vi "SortEngineer.vi"(7 "Invert?":bool, 8 "error in (no error)":errorcluster, 11 "Array in":T1[](array[typedef])) -> (0 "error out":errorcluster, 3 "Array out":T1[](array[typedef]))   [LabVIEW 2017, in "Client.lvlib" / "ParserSorter.lvlib"]
doc: "Check If Days Open > 0,1 and calculate Score based on Prio specific Base Values"
uses:
  ParserSorter.lvlib
  SR Data.ctl
  AE Group.ctl
  SR Status.ctl
  SR Level.ctl
  SR Type.ctl
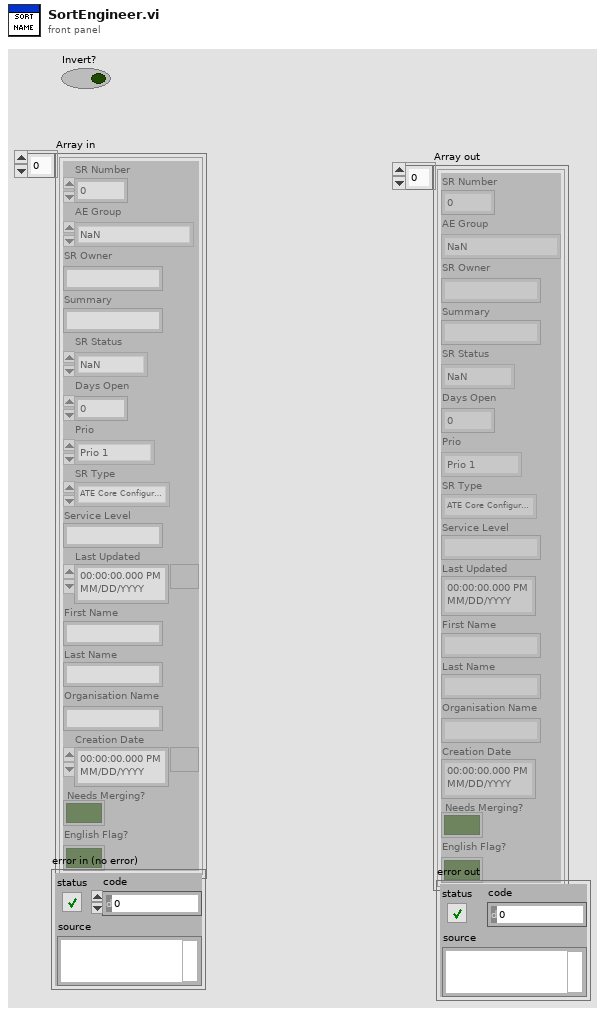
[diagram p1: front panel]
types:
  T1 = typedef "Client.lvlib/ParserSorter.lvlib/SR Data.ctl" = cluster{"SR Number":i64, "AE Group":T2, "SR Owner":string, "Summary":string, "SR Status":T3, "Days Open":dbl, "Prio":T4, "SR Type":T5, "Service Level":string, "Last Updated":timestamp, "First Name":string, "Last Name":string, "Organisation Name":string, "Creation Date":timestamp, "Needs Merging?":bool, "English Flag?":bool}
  T2 = typedef "Client.lvlib/ParserSorter.lvlib/AE Group.ctl" = enum32{"NaN", "AE-Germany", "AE-Poland", "AE-Switzerland", "AE-Czech Republic", "AE-Hungary", "AE-Romania", "AE-Slovakia", "AE-Slovenia"}
  T3 = typedef "Client.lvlib/ParserSorter.lvlib/SR Status.ctl" = enum32{"NaN", "Caller Abandoned", "Created in Error", "Declined to Purchase Support", "Expired", "Forum Resolved AE", "Forum Resolved Customer", "IN WORK", "IN WORK Collab with AES", "IN WORK Collab with PSE", "IN WORK Collab with SE", "IN WORK Escalation", "IN WORK Customer Added Note", "Open", "Potentially Resolved", "POC Resolved", "Resolved", "RMA Waiting on Customer", "RMA Open", "RMA In Progress", "RMA Closed - DOA", "RMA Closed", "RMA Approved for Return", "Project Complete", "Presumed Resolved", "IN WORK Wait on Customer"}
  T4 = typedef "Client.lvlib/ParserSorter.lvlib/SR Level.ctl" = enum16{"Prio 1", "Prio 2", "Prio 3", "Prio 4"}
  T5 = typedef "Client.lvlib/ParserSorter.lvlib/SR Type.ctl" = enum32{"NaN", "ATE Core Configurations (BYOATE)", "Activation", "BioBench", "CAN", "CM C Series", "Calibration", "Consulting Services", "CounterTimer", "DAQExpress", "DASYLab", "DIAdem", "DMM", "DSA HW", "Digital_IO", "FIRST (NIC Only)", "FieldBus", "FieldPoint", "Functional Savety", "GATI", "GPIB", "HMI and Industrial PCs", "HiQ", "HighSpeedDigital_IO", "IMAQ", "IOTech Vibration", "Industrial Communications", "InsightCM", "LV", "LV CD&Sim", "LV Comms", "LV Controls Add-Ons", "LV Embedded", "LV MathScript RT", "LV NXG", "LV NXT", "LVDSC", "LVFPGA", "LVPDA and LV Touch Panel", "LVRT", "LabWindows_CVI", "Lookout", "MATRIXx", "MStudioDotNet", "MStudioVisualBasic", "MStudioVisualC", "Measure (Legacy)", "Motion", "MultifunctionDAQ", "Multimedia Test HW/SW", "Multisim (EWB)", "NI Update Service", "OPC Servers", "Optical (OSI)", "PXI Controllers, Chassis, MXI", "PXI Timing and Sync", "Power Supplies and SMUs", "Powertrain Controls", "RAID", "RF", "RF Software", "RIO", "SC Express", "SCC", "SCXI", "SPEEDY-33 (Hyperception)", "STS", "ScopeDigitizers", "Serial", "Signal Sources", "SignalCondOther", "SignalExpress", "Software Defined Intruments", "Sound and Vibration SW", "Switch Executive", "Switches", "TestStand", "USRP", "Ultiboard (EWB)", "VBench", "VI Logger", "VXI_MXI", "VeriStand", "VisionSW", "VolumeLicenseMgr", "WSN", "Web UI Builder", "myRIO"}
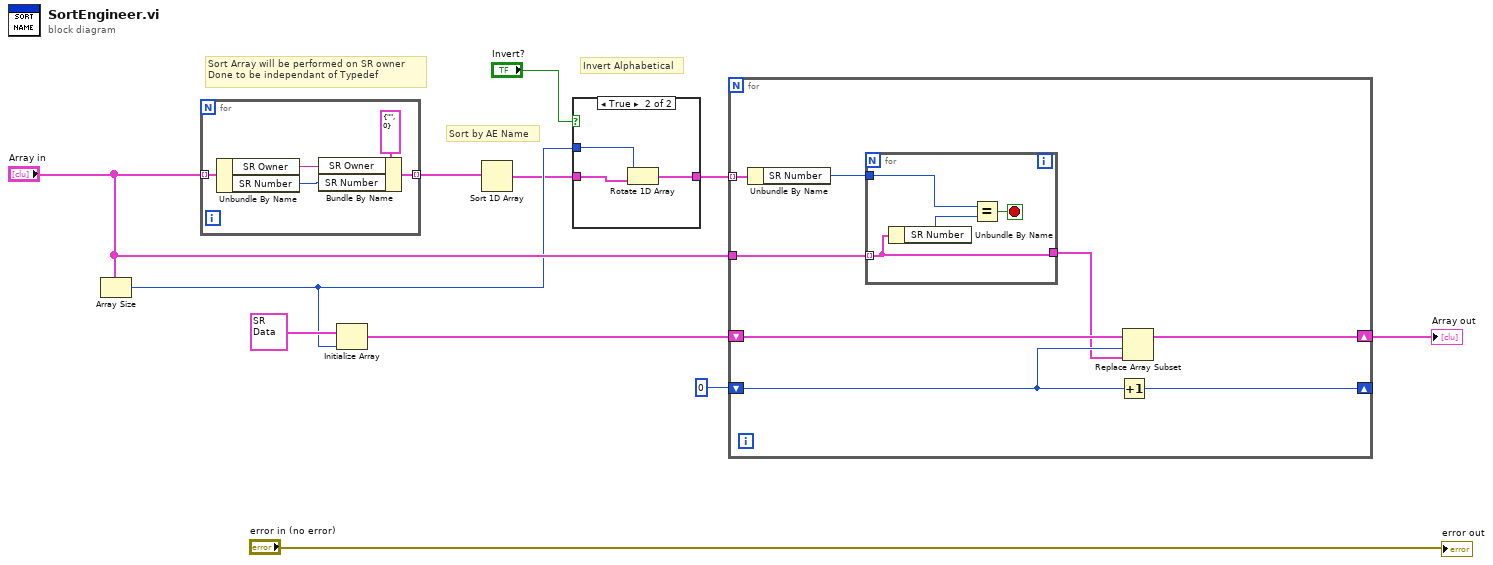
[diagram p0: block diagram]
diagram:
  # "Invert Alphabetical"
  # "Sort Array will be performed on SR owner\nDone to be independant of Typedef"
  # "Sort by AE Name"
  n1 = Array Size(array="Array in") -> (size(s)=w4:i32)
  n2 = for {
    tunnel: "Array in" -> [w16] mode=indexing
    tunnel: [w12] -> w11 mode=indexing
    n3 = Unbundle By Name(w16) -> ("SR Owner"=w14:string, "SR Number"=w13:i64)
    n4 = Bundle By Name(cluster=cluster{"SR Owner":string, "SR Number":i64} {"SR Owner"="", "SR Number"=0}, "SR Owner"=w14, "SR Number"=w13) -> (w12:cluster{"SR Owner":string, "SR Number":i64})
  }
  n5 = Initialize Array(T1 {"SR Number"=0, "AE Group"=enum."NaN", "SR Owner"="", "Summary"="", "SR Status"=enum."NaN", "Days Open"=0.0, "Prio"=enum."Prio 1", "SR Type"=enum."ATE Core Configurations (BYOATE)", "Service Level"="", "Last Updated"=timestamp(0 s since 1904-01-01), "First Name"="", "Last Name"="", "Organisation Name"="", "Creation Date"=timestamp(0 s since 1904-01-01), "Needs Merging?"=FALSE, "English Flag?"=FALSE} ("SR Number"), w4) -> (w8:T1[])
  n6 = Sort 1D Array(array=w11) -> (sorted array=w3:cluster{"SR Owner":string, "SR Number":i64}[])
  n7 = case shown="True" "Invert?" {
    tunnel: w4 -> [_ w20]
    tunnel: w3 -> [w17 w19]
    tunnel: [w17 w18] -> w2
    frame False {
    }
    frame True {
      n8 = Rotate 1D Array(1:w19, 2:w20) -> (0:w18:cluster{"SR Owner":string, "SR Number":i64}[])
    }
  }
  n9 = for {
    tunnel: w2 -> [w28] mode=indexing
    tunnel: "Array in" -> [w27]
    shift-right: [w24] -> w6
    shift-left: w8 -> [w25]
    shift-right: [w22] -> _
    shift-left: 0 ("size(s)") -> [w23]
    n10 = Unbundle By Name(w28) -> ("SR Number"=w26:i64)
    n11 = for {
      tunnel: w27 -> [w29] mode=indexing
      tunnel: w26 -> [w32]
      tunnel: [w29] -> w21
      stop <- w30 stop-if-true
      n12 = Unbundle By Name(w29) -> ("SR Number"=w31:i64)
      n13 = Equal?(x=w32, y=w31) -> (x = y?=w30:bool)
    }
    n14 = Increment(x=w23) -> (x+1=w22:i32)
    n15 = Replace Array Subset(array=w25, new element=w21, index=w23) -> (w24:T1[])
  }
  "Array out" <- w6
  "error out" <- "error in (no error)"
